vi "WeatherMapAPI_CurrentWeather-GetCurrentWeatherData.vi"(8 "error in (no error)":errorcluster) -> (0 "error out":errorcluster, 1 "URL":string, 3 "WeatherMap Current Weather Data":T1)   [LabVIEW 2020]
doc: "Developed By: J Branch\nLast Update: 9/4/2022\n\nDescription: Returns the current weather data to the front panel using the WeatherMap API via HTTP request. The user will need to first navigate to https://openweathermap.org to create an account to get an API key to use the program.\n\nInputs: Zip Code, Country Code\n\nOutput: WeatherMap Current Weather Data Cluster\n\nTo Run: On the block diagram enter the user's API Key into the string text box labelled API Key. Enter the Zip Code and Country Code (us default) in the front panel and select GET Data to execute the API call, the API JSON response will be parsed in the background inside the sub-VIs and formatted to populate the WeatherMap Current Weather Data cluster. \n\nThe Zip Code and County Code can be modified during run-time. \n\nSelect QUIT to terminate the program."
uses:
  <vilib>/httpClient/LabVIEWHTTPClient.lvlib
panel:
  in  "Tab Control":enum32{"User Params", "Internal Params"}(tab)
  out "UserMsg":string
  in  "GetDataButton":bool
  in  "QuitProgramButton":bool
  in  "Zip Code":string
  in  "Country Code":string="us"
  out "HTTP Headers":string
  out "HTTP Body":string
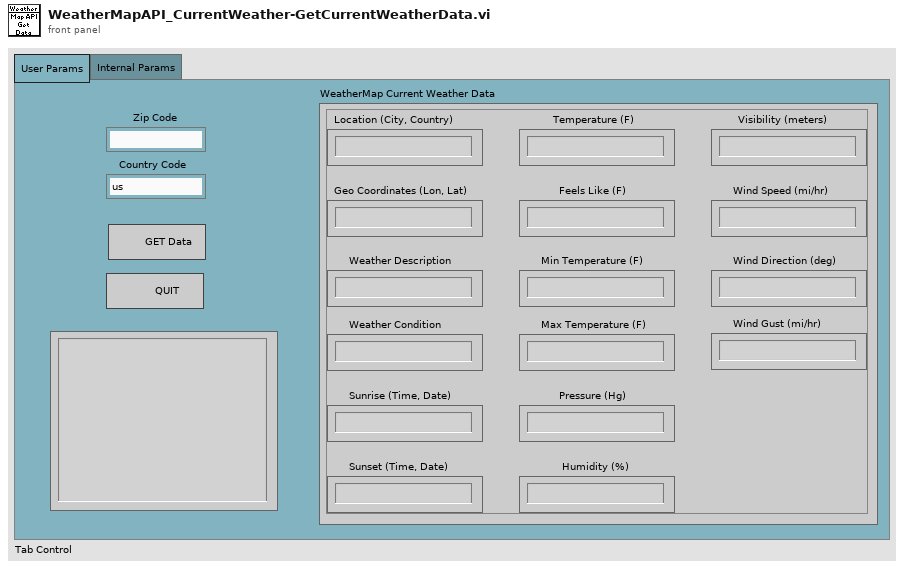
[diagram p1: front panel]
types:
  T1 = cluster{"Location (City, Country)":string, "Geo Coordinates (Lon, Lat)":string, "Weather Description ":string, "Weather Condition":string, "Temperature (F)":string, "Feels Like (F)":string, "Min Temperature (F)":string, "Max Temperature (F)":string, "Pressure (Hg) ":string, "Humidity (%)":string, "Visibility (meters)":string, "Wind Speed (mi/hr)":string, "Wind Direction (deg)":string, "Sunrise (Time, Date)":string, "Sunset (Time, Date)":string, "Wind Gust (mi/hr) ":string}
  T2 = enum8{"Enabled", "Disabled", "Disabled and Grayed Out"}
  T3 = typedef "LabVIEWHTTPClient.lvlib/ClientHandle.ctl" = refnum<k1>
  T4 = cluster{"[0]":string, "[1]":string, "[2]":string, "[3]":string, "[4]":string, "[5]":string, "[6]":string, "[7]":string, "[8]":string, "[9]":string, "[10]":string, "[11]":string, "[12]":string, "[13]":string, "[14]":string, "[15]":string}
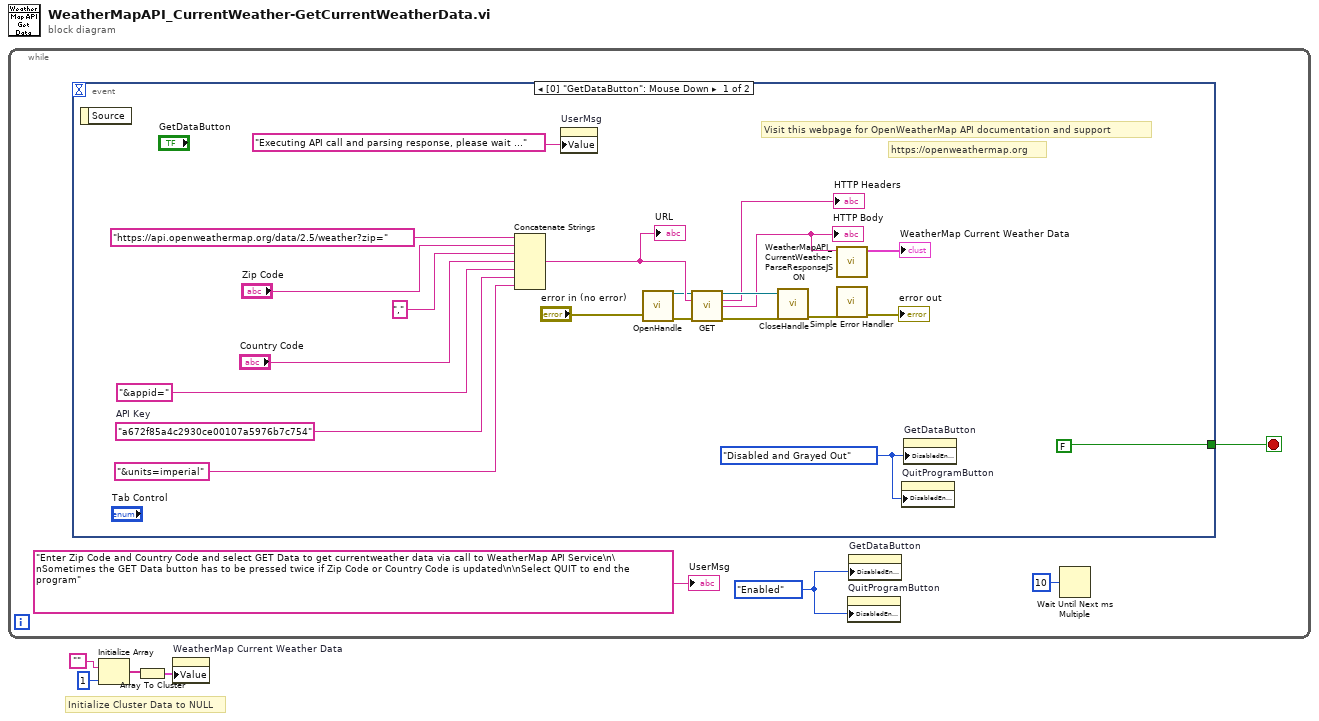
[diagram p0: block diagram]
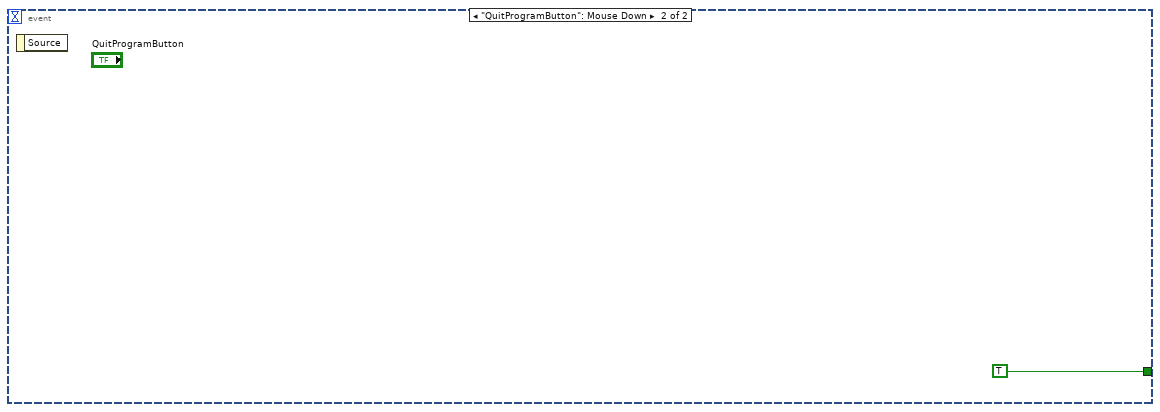
[diagram p2: hidden frame]
diagram:
  # "Initialize Cluster Data to NULL"
  n1 = while {
    stop <- w6 stop-if-true
    w5 = T2."Enabled" ("Disabled")
    n2 = event shown="[0] \"GetDataButton\": Mouse Down" {
      selector: _ -> [_ _]
      dyn-events: _ -> [_ _]
      timeout: _ -> [_ _]
      tunnel: [FALSE TRUE] -> w6
      event "GetDataButton": Mouse Down {
        w17 = T2."Disabled and Grayed Out" ("Disabled")
        w25 = "a672f85a4c2930ce00107a5976b7c754"  # API Key
        # "Visit this webpage for OpenWeatherMap API documentation and support"
        # "https://openweathermap.org"
        n3 = event-data() -> ()  [unwired: 1 in, 1 out]
        n4 = Concatenate Strings("https://api.openweathermap.org/data/2.5/weather?zip=", "Zip Code", ",", "Country Code", "&appid=" ("API Key"), w25, "&units=imperial" ("API Key")) -> (w23:string)
        "URL" <- w23
        n5 = property on="UserMsg" class="Str"("Value"="Executing API call and parsing response, please wait ...") -> ()  [unwired: 2 in, 2 out]
        n6 = call <vilib>:"OpenHandle.vi"("error in (no error)"="error in (no error)") -> ("client handle out"=w16:T3, "error out"=w15:errorcluster)  [unwired: 13 in]
        n7 = call <vilib>:"GET.vi"("client handle"=w16, "url"=w23, "error in (no error)"=w15) -> ("client handle out"=w14:T3, "headers"=→"HTTP Headers":string, "body"=w10:string, "error out"=w13:errorcluster)  [unwired: 9 in]
        "HTTP Body" <- w10
        n8 = call <vilib>:"CloseHandle.vi"("client handle"=w14, "error in (no error)"=w13) -> ("error out"=w11:errorcluster)  [unwired: 13 in]
        n9 = call "WeatherMapAPI_CurrentWeather-ParseResponseJSON.vi"("API JSON Response"=w10) -> ("WeatherMap Current Weather Data"=→"WeatherMap Current Weather Data":T1)  [unwired: 10 in]
        n10 = call <vilib>:"Simple Error Handler.vi"("error in (no error)"=w11) -> ("error out"=→"error out":errorcluster)  [unwired: 4 in, 4 out]
        n11 = property on="QuitProgramButton" class="Bool"("DisabledEnum"=w17) -> ()  [unwired: 2 in, 2 out]
        n12 = property on="GetDataButton" class="Bool"("DisabledEnum"=w17) -> ()  [unwired: 2 in, 2 out]
      }
      event "QuitProgramButton": Mouse Down {
        n13 = event-data() -> ()  [unwired: 1 in, 1 out]
      }
    }
    n14 = property on="QuitProgramButton" class="Bool"("DisabledEnum"=w5) -> ()  [unwired: 2 in, 2 out]
    n15 = property on="GetDataButton" class="Bool"("DisabledEnum"=w5) -> ()  [unwired: 2 in, 2 out]
    n16 = Wait Until Next ms Multiple(millisecond multiple=u32 10) -> ()  [unwired: 1 out]
    "UserMsg" <- "Enter Zip Code and Country Code and select GET Data to get currentweather data via call to WeatherMap API Service\n\nSometimes the GET Data button has to be pressed twice if Zip Code or Country Code is updated\n\nSelect QUIT to end the program" ("String")
  }
  n17 = Initialize Array("", 1 ("dimension size")) -> (w2:string[])
  n18 = Array To Cluster(array=w2) -> (cluster=w1:T4)
  n19 = property on="WeatherMap Current Weather Data" class="Clust (strict)"("Value"=w1) -> ()  [unwired: 2 in, 2 out]
